vi "Bool Decoder.vi"(7 "Optional":bool, 8 "error in (no error)":errorcluster, 9 "Array":u8[](array[numeric]) format="%02x", 10 "Key":i32=-1) -> (0 "error out":errorcluster, 1 "array w/ subset deleted":u8[](array[numeric]) format="%02x", 2 "Read Key":i32, 3 "bool":bool)   [LabVIEW 2016]
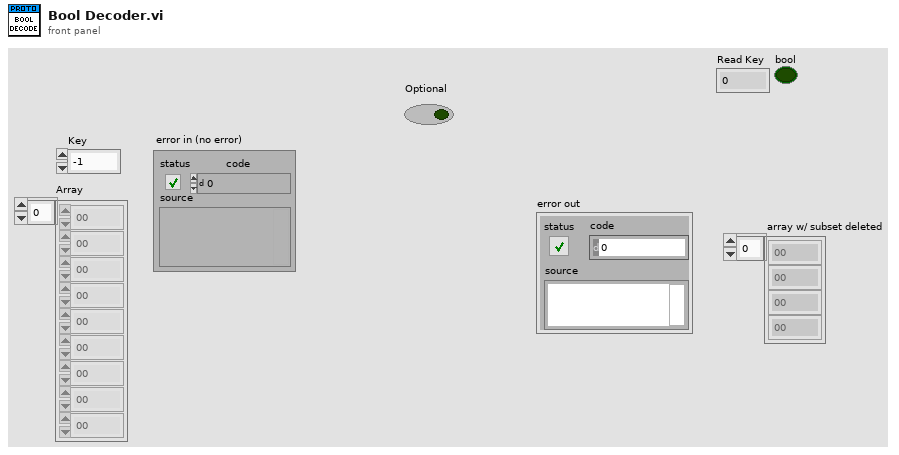
[diagram p1: front panel]
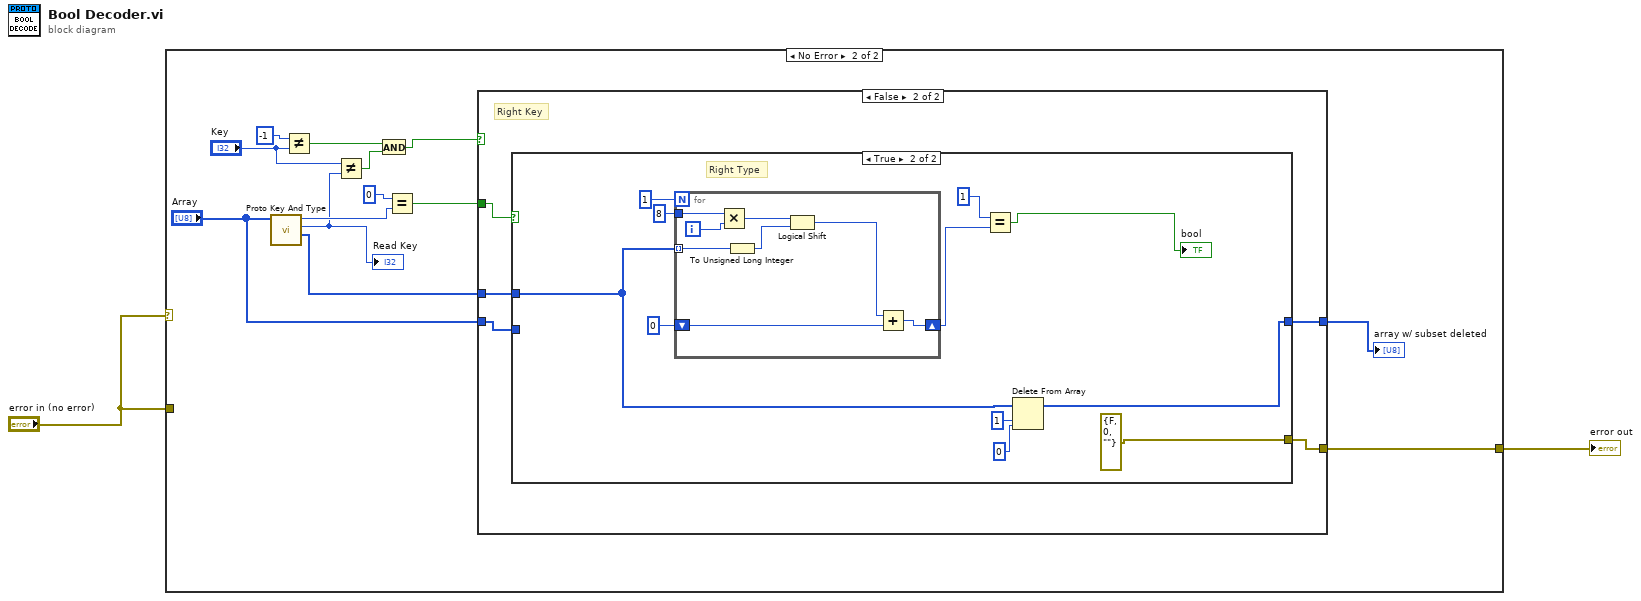
[diagram p0: block diagram]
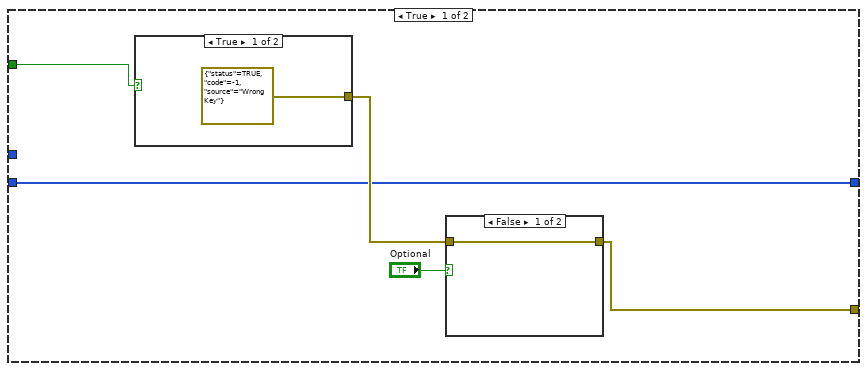
[diagram p3: hidden frame]
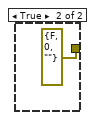
[diagram p4: hidden frame]
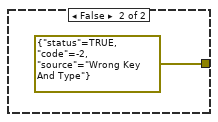
[diagram p5: hidden frame]
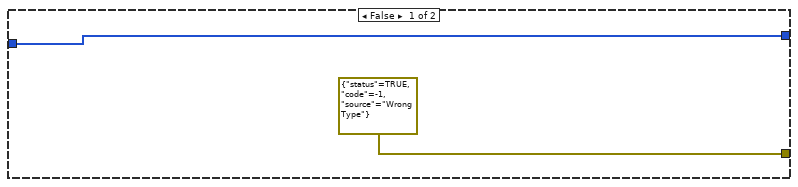
[diagram p6: hidden frame]
diagram:
  n1 = case shown="No Error" "error in (no error)" {
    tunnel: [w3 w4] -> w1
    tunnel: "error in (no error)" -> [w3 _]
    frame Error {
    }
    frame No Error {
      n2 = call "Proto Key And Type.vi"("Array"="Array") -> ("array w/ subset deleted"=w7:u8[], "Key"=w10:i32, "Type"=w11:i32)  [unwired: 8 in]
      "Read Key" <- w10
      n3 = Not Equal?(x=-1, y="Key") -> (x != y?=w15:bool)
      n4 = Not Equal?(x="Key", y=w10) -> (x != y?=w13:bool)
      n5 = And(x=w15, y=w13) -> (x .and. y?=w9:bool)
      n6 = Equal?(x=0, y=w11) -> (x = y?=w8:bool)
      n7 = case shown="False" w9 {
        tunnel: [w19 w30] -> w4
        tunnel: w8 -> [w18 w29]
        tunnel: w7 -> [_ w28]
        tunnel: "Array" -> [w17 w27]
        tunnel: [w17 w26] -> w5
        frame True {
          n8 = case shown="True" w18 {
            tunnel: [errorcluster {"status"=TRUE, "code"=-1, "source"="Wrong Key"} ("error in (no error)") errorcluster {"status"=TRUE, "code"=-2, "source"="Wrong Key And Type"} ("error in (no error)")] -> w20
            frame True {
            }
            frame False {
            }
          }
          n9 = case shown="False" "Optional" {
            tunnel: w20 -> [w22 _]
            tunnel: [w22 errorcluster {"status"=FALSE, "code"=0, "source"=""} ("error in (no error)")] -> w19
            frame False {
            }
            frame True {
            }
          }
        }
        frame False {
          # "Right Key"
          n10 = case shown="True" w29 {
            tunnel: [errorcluster {"status"=TRUE, "code"=-1, "source"="Wrong Type"} ("error in (no error)") errorcluster {"status"=FALSE, "code"=0, "source"=""} ("error in (no error)")] -> w30
            tunnel: w28 -> [_ w36]
            tunnel: w27 -> [w31 _]
            tunnel: [w31 w40] -> w26
            frame False {
            }
            frame True {
              # "Right Type"
              n11 = for {
                N: 1 -> [_]
                tunnel: w36 -> [w45] mode=indexing
                shift-right: [w51] -> w35
                shift-left: 0 -> [w46]
                tunnel: 8 -> [w49]
                i -> [w50]
                n12 = Multiply(x=w49, y=w50) -> (x*y=w48:i32)
                n13 = To Unsigned Long Integer(number=w45) -> (unsigned 32bit integer=w44:u32)
                n14 = Logical Shift(y=w48, x=w44) -> (x << y=w47:u32)
                n15 = Add(x=w47, y=w46) -> (x+y=w51:u32)
              }
              n16 = Equal?(x=u32 1, y=w35) -> (x = y?=→"bool":bool)
              n17 = Delete From Array(array=w36, length=1, index=0) -> (array with subset deleted=w40:u8[])  [unwired: 1 out]
            }
          }
        }
      }
      "array w/ subset deleted" <- w5
    }
  }
  "error out" <- w1
